vi "SpecificProjectType.vi"(8 "error in (no error)":errorcluster, 10 "Action":enum16{"Clear", "Get", "Set"}(ring), 11 "MetaDataObj in":refnum<class "MetaDataObj.lvclass">) -> (0 "error out":errorcluster, 1 "Project Name":string, 2 "Project Root":path, 3 "MetaDataObj out":refnum<class "MetaDataObj.lvclass">)   [LabVIEW 2021, in "myRIOMetaDataObj.lvclass"]
uses:
  myRIOMetaDataObj.lvclass
  <resource>/dialog/NewProjectWizard/MetaDataObj/MetaDataObj.lvclass
  p:/lvdist/win32/export/21.0/21.0.0f0/dist/resource/dialog/NewProjectWizard/MetaDataObj/MetaDataObj.lvclass
  <resource>/dialog/NewProjectWizard/MetaDataObj/Accessors/Read Project Path.vi
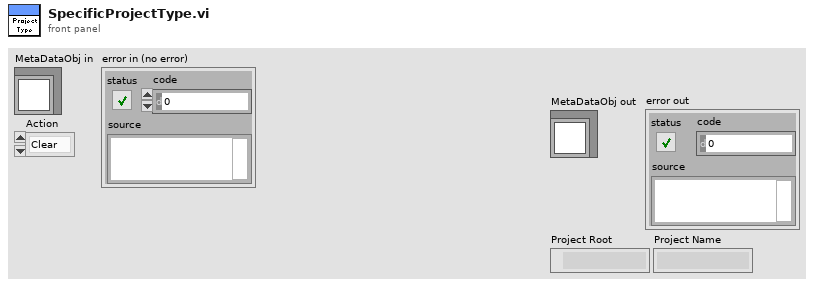
[diagram p1: front panel]
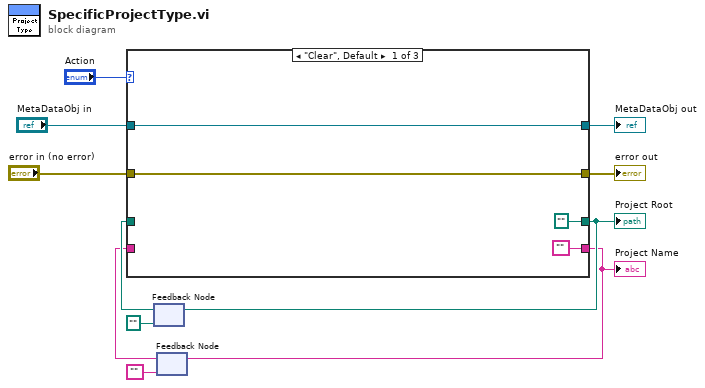
[diagram p0: block diagram]
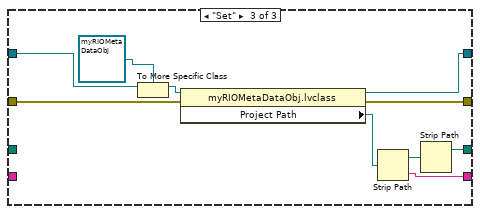
[diagram p3: hidden frame]
diagram:
  n1 = feedback #1(path "") -> (w5:path)
  n2 = feedback #2("") -> (w2:string)
  n3 = case shown="\"Clear\", Default" "Action" {
    tunnel: "MetaDataObj in" -> [w15 w19 w27]
    tunnel: [w15 w19 w26] -> w9
    tunnel: "error in (no error)" -> [w14 w18 w25]
    tunnel: [w14 w18 w24] -> w7
    tunnel: [path "" w17 w21] -> w6
    tunnel: w5 -> [_ w17 _]
    tunnel: ["" w16 w20] -> w3
    tunnel: w2 -> [_ w16 _]
    frame "Clear", Default {
    }
    frame "Get" {
    }
    frame "Set" {
      n4 = To More Specific Class(target class=refnum<class "myRIOMetaDataObj.lvclass"> refnum ("myRIOMetaDataObj.lvclass"), reference=w27) -> (specific class reference=w29:refnum<class "myRIOMetaDataObj.lvclass">)  [unwired: 1 in, 1 out]
      n5 = property class="myRIOMetaDataObj.lvclass"(reference=w29, error in=w25) -> (reference out=w26:refnum<class "myRIOMetaDataObj.lvclass">, error out=w24:errorcluster, "Project Path"=w23:path)
      n6 = Strip Path(path=w23) -> (stripped path=w22:path, name=w20:string)
      n7 = Strip Path(path=w22) -> (stripped path=w21:path)  [unwired: 1 out]
    }
  }
  "MetaDataObj out" <- w9
  "error out" <- w7
  "Project Root" <- w6
  "Project Name" <- w3
  n8 = feedback-in #1(w6) -> ()
  n9 = feedback-in #2(w3) -> ()
